vi "roboRIO v1.0 Write Relay.vi"(8 "error in (no error)":errorcluster, 9 "Relay Values List":T1[](array[typedef]), 10 "Channel List":T4, 11 "myRIO Ref In":T2) -> (0 "error out":errorcluster, 3 "myRIO Ref Out":T2)   [LabVIEW 2021]
uses:
  <vilib>/myRIO/Common/Instrument Driver Framework/roboRIO v1.0/Relay/typedefs/Relay Channels List.ctl
  <vilib>/myRIO/Common/Instrument Driver Framework/roboRIO v1.0/Relay/typedefs/Relay Channels Enum.ctl
  <vilib>/myRIO/Common/Instrument Driver Framework/Utilities/typedefs/myRIO v1.0 Reference.ctl
  <vilib>/myRIO/Common/Instrument Driver Framework/Utilities/typedefs/Generic FPGA Reference.ctl
  <vilib>/myRIO/Common/Instrument Driver Framework/roboRIO v1.0/Relay/typedefs/Relay Value.ctl
  <vilib>/myRIO/Common/Instrument Driver Framework/roboRIO v1.0/Relay/typedefs/Relay FPGA Reference.ctl
  <vilib>/rvi/errors/niLvFpgaAdjustHostInterfaceError.vi
  <vilib>/rvi/interface/nirviReadWriteControl/nirviReadWriteControl.xnode
  <vilib>/rvi/interface/Simulation/niFpgaSimulationCallBeginRW.vi
  NiFpgaLv.dll
panel:
  # "This VI writes boolean values to a user specified a list of DIO channels on the myRIO v1.0 hardware. The value is input as a boolean value. Please see Block Diagram for details."
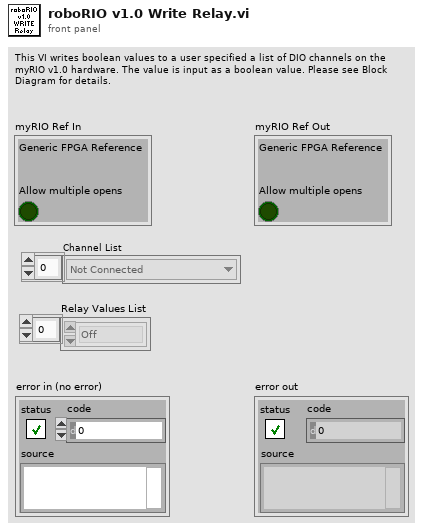
[diagram p1: front panel]
types:
  T1 = typedef "Relay Value.ctl" = enum16{"Off", "On", "Forward", "Reverse"}
  T2 = typedef "myRIO v1.0 Reference.ctl" = cluster{"Generic FPGA Reference":T3, "Allow multiple opens":bool}
  T3 = typedef "Generic FPGA Reference.ctl" = refnum<k20>
  T4 = typedef "Relay Channels List.ctl" = T5[]
  T5 = typedef "Relay Channels Enum.ctl" = enum16{"Not Connected", "RELAY/RELAY0", "RELAY/RELAY1", "RELAY/RELAY2", "RELAY/RELAY3"}
  T6 = typedef "Relay FPGA Reference.ctl" = refnum<k20>
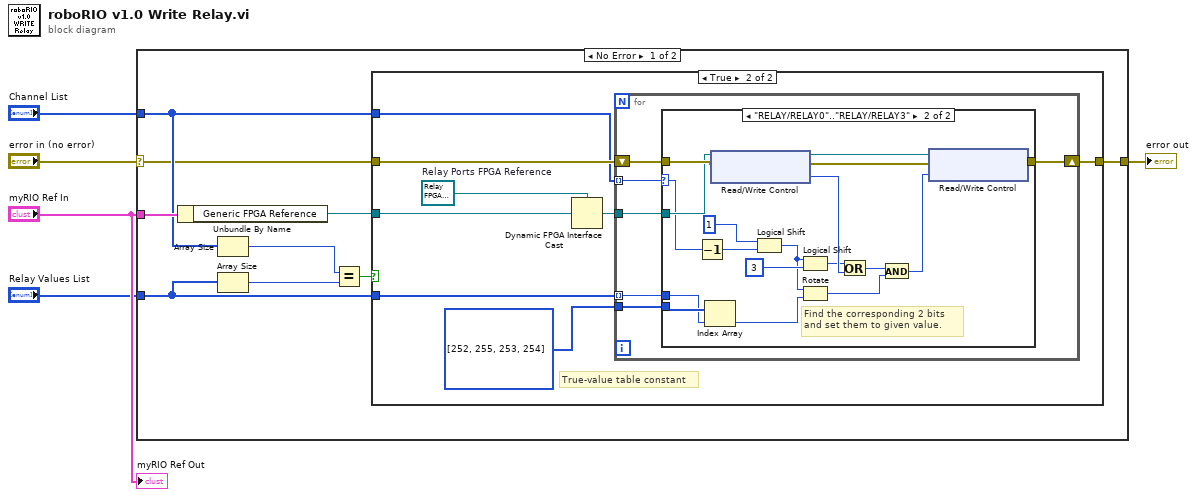
[diagram p0: block diagram]
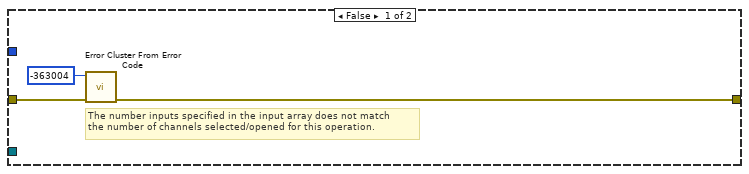
[diagram p2: hidden frame]
diagram:
  n1 = case shown="No Error" "error in (no error)" {
    selector: "error in (no error)" -> [w7 w51]
    tunnel: "myRIO Ref In" -> [w14 _]
    tunnel: [w13 w51] -> w4
    tunnel: "Channel List" -> [w10 _]
    tunnel: "Relay Values List" -> [w9 _]
    frame No Error {
      n2 = Unbundle By Name(w14) -> ("Generic FPGA Reference"=w6:T3)
      n3 = Array Size(array=w10) -> (size(s)=w12:i32)
      n4 = Array Size(array=w9) -> (size(s)=w11:i32)
      n5 = Equal?(x=w12, y=w11) -> (x = y?=w8:bool)
      n6 = case shown="True" w8 {
        tunnel: w10 -> [_ w20]
        tunnel: w9 -> [_ w19]
        tunnel: w6 -> [_ w24]
        tunnel: w7 -> [w16 w22]
        tunnel: [w15 w21] -> w13
        frame False {
          # "The number inputs specified in the input array does not match\nthe number of channels selected/opened for this operation."
          n7 = call <vilib>:"Error Cluster From Error Code.vi"("error in (no error)"=w16, "error code (0)"=-363004) -> ("error out"=w15:errorcluster)  [unwired: 7 in]
        }
        frame True {
          w25 = T6 refnum  # Relay Ports FPGA Reference
          # "True-value table constant"
          n8 = Dynamic FPGA Interface Cast(Session In=w25, Type=w24) -> (Session Out=w23:T6)
          n9 = for {
            tunnel: w23 -> [w31]
            tunnel: w20 -> [w28] mode=indexing
            shift-right: [w29] -> w21
            shift-left: w22 -> [w30]
            tunnel: w19 -> [w27] mode=indexing
            tunnel: u8[] [252, 255, 253, 254] -> [w26]
            n10 = case shown="\"RELAY/RELAY0\"..\"RELAY/RELAY3\"" w28 {
              selector: w28 -> [_ w42]
              tunnel: w31 -> [_ w47]
              tunnel: w30 -> [w32 w49]
              tunnel: [w32 w50] -> w29
              tunnel: w27 -> [_ w37]
              tunnel: w26 -> [_ w38]
              frame "Not Connected", Default {
              }
              frame "RELAY/RELAY0".."RELAY/RELAY3" {
                # "Find the corresponding 2 bits and set them to given value."
                n11 = Decrement(x=w42) -> (x-1=w43:T5)
                n12 = Index Array(array=w38, index=w37) -> (element=w36:u8)
                n13 = xnode "Read/Write Control"("FPGA VI Reference In"=w47, "error in"=w49) -> ("FPGA VI Reference Out"=w46:T6, "error out"=w48:errorcluster, "DO.RELAY.OUT"=w41:u8)
                n14 = Logical Shift(y=i16 1, x=w43) -> (x << y=w39:u32)
                n15 = Logical Shift(y=w39, x=u8 3) -> (x << y=w40:u8)
                n16 = Rotate(1:w36, 2:w39) -> (0:w34:u8)
                n17 = Or(x=w40, y=w41) -> (x .or. y?=w35:u8)
                n18 = And(x=w35, y=w34) -> (x .and. y?=w33:u8)
                n19 = xnode "Read/Write Control"("FPGA VI Reference In"=w46, "error in"=w48, "DO.RELAY.OUT"=w33) -> ("error out"=w50:errorcluster)  [unwired: 1 out]
              }
            }
          }
        }
      }
    }
    frame Error {
    }
  }
  "error out" <- w4
  "myRIO Ref Out" <- "myRIO Ref In"
